vi "LAKESHORE_8_01_2023.vi"() -> ()   [LabVIEW 2020]
panel:
  in  "Select Parameter":enum16{"Resistance(ohms)", "Temperature(K)"}(ring)
  in  "Channel":string
  out "XY Graph":cluster{"X":dbl[], "Y":dbl[]}[](graph)
  out "Measured Value":dbl
  in  "VISA resource name":refnum<visa-resource-name>
  # "LAKE SHORE"
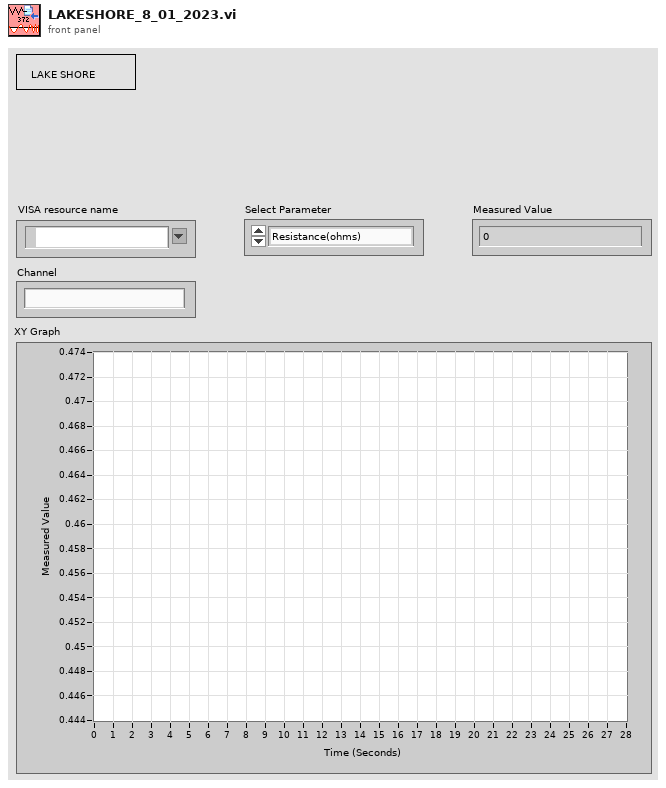
[diagram p1: front panel]
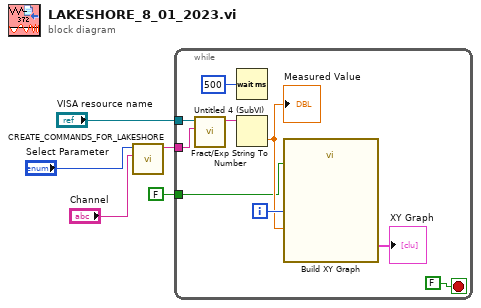
[diagram p0: block diagram]
diagram:
  n1 = call "CREATE_COMMANDS_FOR_LAKESHORE.vi"("Channel"="Channel", "Select Parameter"="Select Parameter") -> ("result string"=w4:string)  [unwired: 9 in]
  n2 = while {
    tunnel: "VISA resource name" -> [w13]
    tunnel: w4 -> [w12]
    tunnel: FALSE ("Reset") -> [w7]
    i -> [w9]
    stop <- FALSE stop-if-true
    n3 = call "Untitled 4 (SubVI).vi"("ID Query"=w12, "VISA Refnum in"=w13) -> ("read buffer"=w14:string)  [unwired: 9 in]
    n4 = Wait (ms)(milliseconds to wait=u32 500) -> ()  [unwired: 1 out]
    n5 = Fract/Exp String To Number(string=w14) -> (number=w8:dbl)  [unwired: 3 in, 1 out]
    "Measured Value" <- w8
    n6 = call "Build XY Graph"("Reset"=w7, "Y Input"=w8, "X Input"=w9) -> ("XY Graph"=→"XY Graph":cluster{"X":dbl[], "Y":dbl[]}[])  [unwired: 7 in, 1 out]
  }
